vi "q.vi"(6 "Variant in":variant, 7 "Shift Pressed?":bool, 8 "error in (no error)":errorcluster, 10 "QD Combo Box Ref":refnum<vi>, 11 "QD Launch VI Ref":refnum<vi>) -> (0 "error out":errorcluster, 4 "Variant out":variant)   [LabVIEW 2014]
uses:
  <vilib>/Utility/traverseref.llb/TRef TravTarget.ctl
  <vilib>/Utility/miscctls.llb/LVPoint32TypeDef.ctl
  <vilib>/Utility/inputDevices.llb/mouseAcquire.vi
  <vilib>/Utility/inputDevices.llb/closeMouse.vi
  <vilib>/Utility/VariantDataType/VariantType.lvlib
panel:
  # "Do not change the connector pane of this VI."
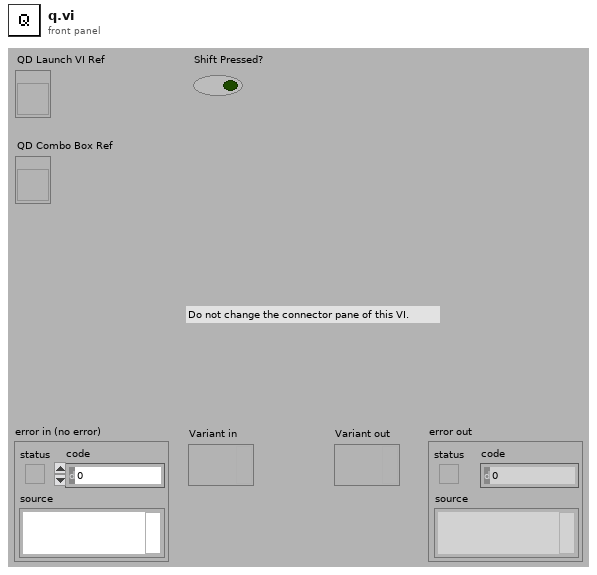
[diagram p1: front panel]
types:
  T1 = typedef "LVPoint32TypeDef.ctl" = cluster{"Horizontal":i32, "Vertical":i32}
  T2 = typedef "TRef TravTarget.ctl" = enum16{"FP", "BD", "Other"}
  T3 = typedef "LVRectTypeDef.ctl" = cluster{"Left":i16, "Top":i16, "Right":i16, "Bottom":i16}
  T4 = typedef "LVPointTypeDef.ctl" = cluster{"Horizontal":i16, "Vertical":i16}
  T5 = cluster{"Horizontal":i32, "Vertical":i32, "Scrolling":i32}
  T6 = typedef "VariantType.lvlib/Type.ctl" = enum8{"Invalid Type", "Void", "I8", "I16", "I32", "I64", "U8", "U16", "U32", "U64", "Single Float", "Double Float", "Extended Float", "Single Complex", "Double Complex", "Extended Complex", "Enum U8", "Enum U16", "Enum U32", "Enum U64", "Single Float With Unit", "Double Float With Unit", "Extended Float With Unit", "Single Complex with Unit", "Double Complex with Unit", "Extended Complex with Unit", "Boolean", "String", "Path", "Picture", "Tag", "Array", "Cluster", "Variant", "LV Variant", "Waveform", "Timestamp", "Digital Waveform", "Digital Data", "ExpressData", "Refnum", "External Data", "VI", "Poly VI", "LabVIEW Class Instance", "Fixed Point"}
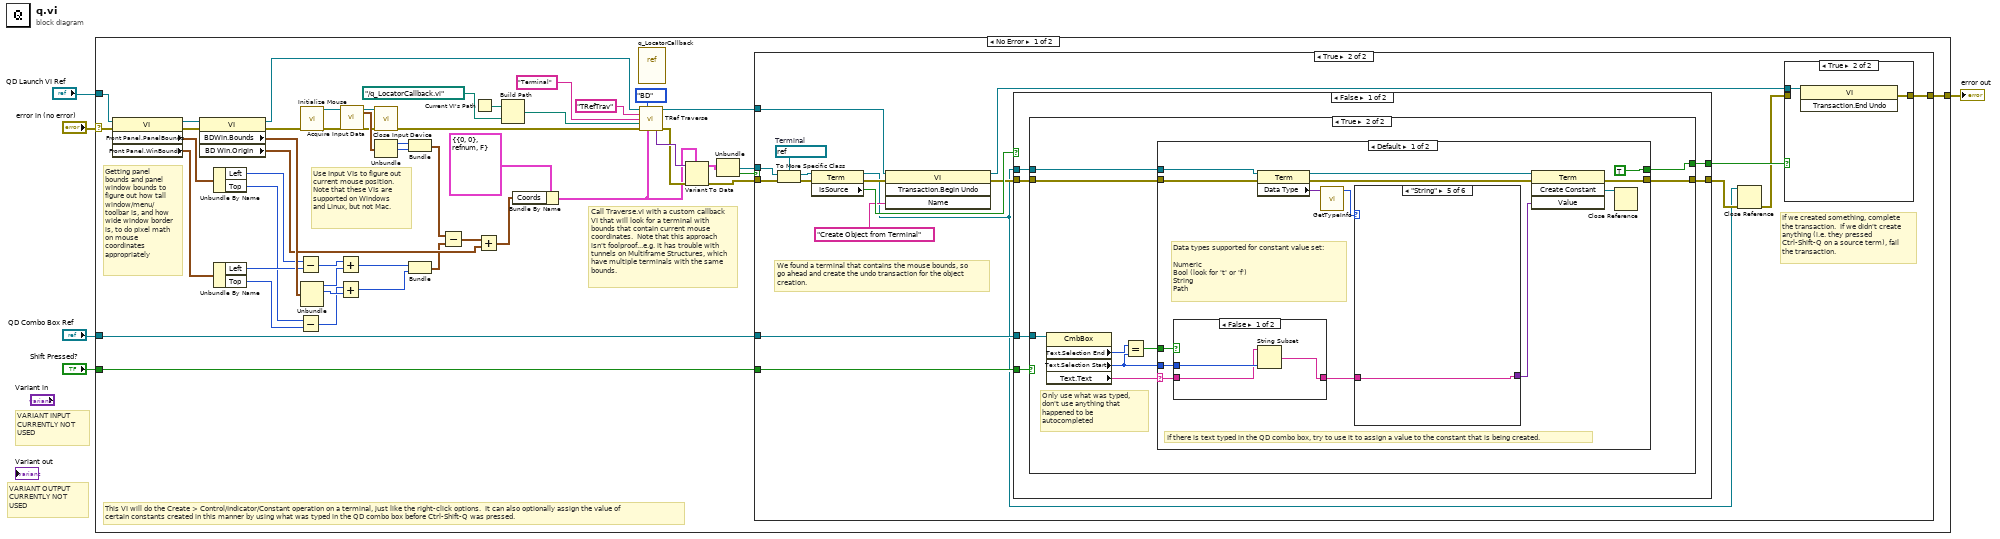
[diagram p0: block diagram]
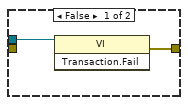
[diagram p3: hidden frame]
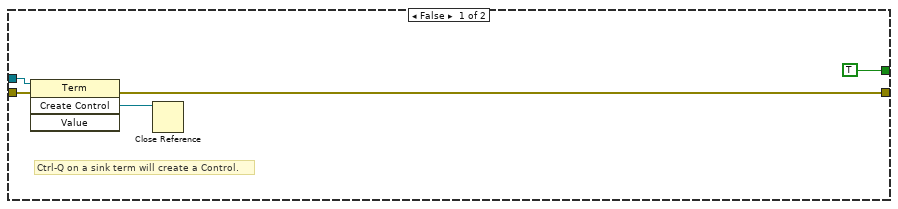
[diagram p4: hidden frame]
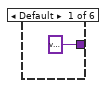
[diagram p5: hidden frame]
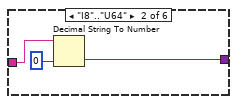
[diagram p6: hidden frame]
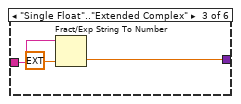
[diagram p7: hidden frame]
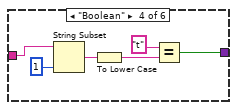
[diagram p8: hidden frame]
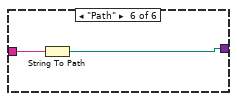
[diagram p9: hidden frame]
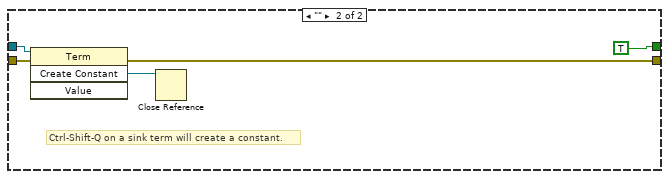
[diagram p11: hidden frame]
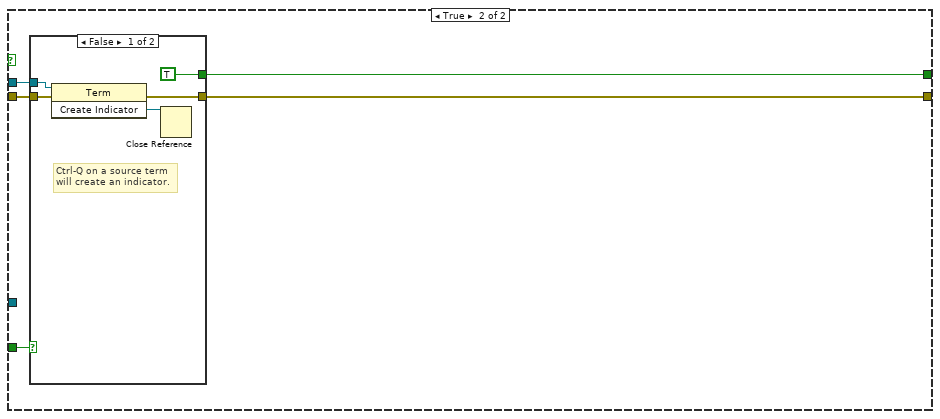
[diagram p12: hidden frame]
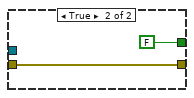
[diagram p13: hidden frame]
diagram:
  # "VARIANT INPUT\nCURRENTLY NOT\nUSED"
  # "VARIANT OUTPUT\nCURRENTLY NOT\nUSED"
  n1 = case shown="No Error" "error in (no error)" {
    selector: "error in (no error)" -> [w23 w150]
    tunnel: [w38 w150] -> w4
    tunnel: "QD Launch VI Ref" -> [w36 _]
    tunnel: "Shift Pressed?" -> [w40 _]
    tunnel: "QD Combo Box Ref" -> [w37 _]
    frame No Error {
      # "This VI will do the Create > Control/Indicator/Constant operation on a terminal, just like the right-click options.  It can also optionally assign the value of certain constants created in this manner by using what was typed in the QD combo box before Ctrl-Shift-Q was pressed."
      # "Call Traverse.vi with a custom callback VI that will look for a terminal with bounds that contain current mouse coordinates.  Note that this approach isn't foolproof...e.g. it has trouble with tunnels on Multiframe Structures, which have multiple terminals with the same bounds."
      # "Use Input VIs to figure out current mouse position.  Note that these VIs are supported on Windows and Linux, but not Mac."
      # "Getting panel bounds and panel window bounds to figure out how tall window/menu/toolbar is, and how wide window border is, to do pixel math on mouse coordinates appropriately"
      n2 = property class="VI"(reference=w36, error in=w23) -> (reference out=w21:refnum<vi>, error out=w22:errorcluster, "Front Panel.PanelBounds"=w35:T3, "Front Panel.WinBounds"=w34:T3)
      n3 = property class="VI"(reference=w21, error in=w22) -> (reference out=w20:refnum<vi>, error out=w39:errorcluster, "BDWin.Bounds"=w55:T3, "BD Win.Origin"=w46:T4)
      n4 = Unbundle By Name(w35) -> ("Left"=w33:i16, "Top"=w30:i16)
      n5 = Unbundle By Name(w34) -> ("Left"=w32:i16, "Top"=w31:i16)
      n6 = Subtract(x=w33, y=w32) -> (x-y=w28:i16)
      n7 = Subtract(x=w30, y=w31) -> (x-y=w25:i16)
      n8 = call <vilib>:"Initialize Mouse.vi"("error in (no error)"=w39) -> ("error out"=w50:errorcluster, "device ID"=w49:refnum<k1>)  [unwired: 9 out]
      n9 = Unbundle(w55) -> ("Left"=w29:i16, "Top"=w26:i16)  [unwired: 2 out]
      n10 = Add(x=w28, y=w29) -> (x+y=w27:i16)
      n11 = Add(x=w25, y=w26) -> (x+y=w24:i16)
      n12 = call-poly <vilib>:"Acquire Input Data.vi"("device ID"=w49, "error in (no error)"=w50) -> ("device ID"=w48:refnum<k1>, "axis info"=w51:T5, "error out"=w47:errorcluster)  [unwired: 1 in, 14 out]
      n13 = call-poly <vilib>:"Close Input Device.vi"("error in (no error)"=w47, "device ID"=w48) -> ("error out"=w19:errorcluster)  [unwired: 8 out]
      n14 = Unbundle(w51) -> ("Horizontal"=w52:i32, "Vertical"=w53:i32)  [unwired: 1 out]
      n15 = Bundle("Horizontal"=w52, "Vertical"=w53) -> (w54:cluster{"Horizontal":i32, "Vertical":i32})  [unwired: 1 out]
      n16 = Bundle(w27, w24) -> (w44:cluster{i16, i16})  [unwired: 1 out]
      n17 = Subtract(x=w54, y=w44) -> (x-y=w45:cluster{i32, i32})
      n18 = Current VI's Path() -> (path=w8:path)
      n19 = Add(x=w45, y=w46) -> (x+y=w42:cluster{i32, i32})
      n20 = Build Path(base path=w8, name or relative path=path "../q_LocatorCallback.vi") -> (appended path=w16:path)
      n21 = Bundle By Name(cluster=cluster{"Coords":T1, refnum<vi>, "Found?":bool} {"Coords"={"Horizontal"=0, "Vertical"=0}, refnum, "Found?"=FALSE}, "Coords"=w42) -> (w11:cluster{"Coords":T1, refnum<vi>, "Found?":bool})
      n22 = vi-ref <resource>:"q_LocatorCallback.vi"() -> ()  [unwired: 1 out]
      n23 = call <vilib>:"TRef Traverse.vi"("VI Refnum"=w20, "Traverse Target"=TRef_TravTarget."BD", "OpName (\"TRefTrav\")"="TRefTrav", "Class Name"="Terminal", "Callback Path"=w16, "error in (no error)"=w19, "ContextData type"=w11) -> ("dup VI Refnum"=w18:refnum<vi>, "ContextData"=w17:variant, "error out"=w15:errorcluster)  [unwired: 2 in, 4 out]
      n24 = Variant To Data(error in=w15, type=w11, Variant=w17) -> (data=w13:cluster{"Coords":T1, refnum<vi>, "Found?":bool}, error out=w43:errorcluster)
      n25 = Unbundle(w13) -> (w41:refnum<vi>, "Found?"=w6:bool)  [unwired: 1 out]
      n26 = case shown="True" w6 {
        tunnel: w43 -> [w56 w73]
        tunnel: w41 -> [_ w72]
        tunnel: w40 -> [_ w68]
        tunnel: [w56 w67] -> w38
        tunnel: w37 -> [_ w66]
        tunnel: w18 -> [_ w63]
        frame False {
        }
        frame True {
          w74 = refnum<vi> refnum  # Terminal
          # "If we created something, complete the transaction.  If we didn't create anything (i.e. they pressed Ctrl-Shift-Q on a source term), fail the transaction."
          # "We found a terminal that contains the mouse bounds, so go ahead and create the undo transaction for the object creation."
          n27 = To More Specific Class(target class=w74, reference=w72, error in=w73) -> (specific class reference=w70:refnum<vi>, error out=w71:errorcluster)
          n28 = property class="Term"(reference=w70, error in=w71) -> (reference out=w57:refnum<vi>, error out=w65:errorcluster, "IsSource"=w69:bool)
          n29 = invoke class="VI" method="Transaction.Begin Undo"(reference=w63, error in=w65, "Name"="Create Object from Terminal") -> (reference out=w62:refnum<vi>, error out=w64:errorcluster)  [unwired: 1 in, 2 out]
          n30 = case shown="False" w69 {
            tunnel: [w82 w142] -> w59
            tunnel: w68 -> [w81 w141]
            tunnel: w64 -> [w83 w140]
            tunnel: w57 -> [w84 w139]
            tunnel: w66 -> [w80 _]
            tunnel: [w79 w138] -> w60
            frame False {
              n31 = case shown="True" w81 {
                tunnel: w84 -> [w89 w98]
                tunnel: w83 -> [w88 w96]
                tunnel: [w87 w97] -> w82
                tunnel: w80 -> [_ w92]
                tunnel: [TRUE w90] -> w79
                frame False {
                  # "Ctrl-Q on a sink term will create a Control."
                  n32 = invoke class="Term" method="Create Control"(reference=w89, error in=w88) -> (error out=w87:errorcluster, "Create Control"=w85:refnum<vi>)  [unwired: 2 in, 2 out]
                  n33 = Close Reference(reference=w85) -> ()  [unwired: 1 in, 1 out]
                }
                frame True {
                  # "Only use what was typed, don't use anything that happened to be autocompleted"
                  n34 = property on="Property Node" class="CmbBox"(reference=w92) -> ("Text.Selection End"=w95:u32, "Text.Selection Start"=w93:u32, "Text.Text"=w91:string)  [unwired: 1 in, 2 out]
                  n35 = Equal?(x=w95, y=w93) -> (x = y?=w94:bool)
                  n36 = case shown="Default" w91 {
                    selector: w91 -> [w109 _]
                    tunnel: w98 -> [w107 w137]
                    tunnel: [w112 w136] -> w97
                    tunnel: w96 -> [w108 w135]
                    tunnel: w94 -> [w111 _]
                    tunnel: w93 -> [w110 _]
                    tunnel: [TRUE TRUE] -> w90
                    frame Default {
                      # "Data types supported for constant value set:\n\nNumeric\nBool (look for 't' or 'f')\nString\nPath"
                      # "If there is text typed in the QD combo box, try to use it to assign a value to the constant that is being created."
                      n37 = case shown="False" w111 {
                        tunnel: [w131 w132] -> w102
                        tunnel: w110 -> [w130 _]
                        tunnel: w109 -> [w129 w132]
                        frame False {
                          n38 = String Subset(string=w129, length (rest)=w130) -> (substring=w131:string)  [unwired: 1 out]
                        }
                        frame True {
                        }
                      }
                      n39 = property class="Term"(reference=w107, error in=w108) -> (reference out=w106:refnum<vi>, error out=w105:errorcluster, "Data Type"=w104:variant)
                      n40 = call <vilib>:"GetTypeInfo.vi"("Variant"=w104) -> ("Type Enum"=w103:T6)  [unwired: 6 in, 4 out]
                      n41 = case shown="\"String\"" w103 {
                        tunnel: w102 -> [_ w116 w119 w125 w126 w128]
                        tunnel: [variant ("variant") w115 w117 w120 w126 w127] -> w101
                        frame Default {
                        }
                        frame "I8".."U64" {
                          n42 = Decimal String To Number(string=w116, default (0L)=u64 0) -> (number=w115:u64)  [unwired: 1 in, 1 out]
                        }
                        frame "Single Float".."Extended Complex" {
                          n43 = Fract/Exp String To Number(string=w119, default (0 dbl)=ext 0.0) -> (number=w117:ext)  [unwired: 2 in, 1 out]
                        }
                        frame "Boolean" {
                          n44 = String Subset(string=w125, length (rest)=1 ("length (rest)")) -> (substring=w123:string)  [unwired: 1 in]
                          n45 = To Lower Case(string=w123) -> (all lower case string=w122:string)
                          n46 = Equal?(x="t", y=w122) -> (x = y?=w120:bool)
                        }
                        frame "String" {
                        }
                        frame "Path" {
                          n47 = String To Path(string=w128) -> (path=w127:path)
                        }
                      }
                      n48 = invoke class="Term" method="Create Constant"(reference=w106, error in=w105, "Value"=w101) -> (error out=w112:errorcluster, "Create Constant"=w99:refnum<vi>)  [unwired: 1 in, 2 out]
                      n49 = Close Reference(reference=w99) -> ()  [unwired: 1 in, 1 out]
                    }
                    frame "" {
                      # "Ctrl-Shift-Q on a sink term will create a constant."
                      n50 = invoke class="Term" method="Create Constant"(reference=w137, error in=w135) -> (error out=w136:errorcluster, "Create Constant"=w133:refnum<vi>)  [unwired: 2 in, 2 out]
                      n51 = Close Reference(reference=w133) -> ()  [unwired: 1 in, 1 out]
                    }
                  }
                }
              }
            }
            frame True {
              n52 = case shown="False" w141 {
                tunnel: w139 -> [w147 _]
                tunnel: w140 -> [w145 w149]
                tunnel: [w146 w149] -> w142
                tunnel: [TRUE FALSE] -> w138
                frame False {
                  # "Ctrl-Q on a source term will create an indicator."
                  n53 = invoke class="Term" method="Create Indicator"(reference=w147, error in=w145) -> (error out=w146:errorcluster, "Create Indicator"=w143:refnum<vi>)  [unwired: 1 in, 1 out]
                  n54 = Close Reference(reference=w143) -> ()  [unwired: 1 in, 1 out]
                }
                frame True {
                }
              }
            }
          }
          n55 = Close Reference(reference=w57, error in (no error)=w59) -> (error out=w58:errorcluster)
          n56 = case shown="True" w60 {
            tunnel: [w75 w78] -> w67
            tunnel: w62 -> [w76 w77]
            tunnel: w58 -> [_ _]
            frame False {
              n57 = invoke class="VI" method="Transaction.Fail"(reference=w76) -> (error out=w75:errorcluster)  [unwired: 2 in, 2 out]
            }
            frame True {
              n58 = invoke class="VI" method="Transaction.End Undo"(reference=w77) -> (error out=w78:errorcluster)  [unwired: 2 in, 2 out]
            }
          }
        }
      }
    }
    frame Error {
    }
  }
  "error out" <- w4
